vi "Do.vi"(8 "error in (no error)":errorcluster, 9 "Events":refnum<class "Events.lvclass">, 10 "Message Loop Data in":T1, 11 "IInternalRequest in":refnum<class "RegisteredHandler JSON.lvclass">) -> (0 "error out":errorcluster, 2 "Message Loop Data out":T1, 3 "IInternalRequest out":refnum<class "RegisteredHandler JSON.lvclass">)   [LabVIEW 2020, in "wamplv.lvlib" / "RegisteredHandler JSON.lvclass"]
uses:
  RegisteredHandler JSON.lvclass
  WAMP Client/Private/TypeDef/Publish Requests Map.ctl
  wamplv.lvlib
  WAMP Client/Private/TypeDef/Endpoint Data.ctl
  Call/ICallRequest/ICallRequest.lvclass
  WAMP Client/Private/TypeDef/CALL Request Map.ctl
  WAMP Client/Private/TypeDef/SUBSCRIBE Requests Map.ctl
  WAMP Client/Private/TypeDef/Subscriptions Map.ctl
  WAMP Client/Private/TypeDef/Unsubscribe Requests Map.ctl
  WAMP Client/Private/TypeDef/Unregister requests map.ctl
  WAMP Client/Private/TypeDef/Message Loop Data.ctl
  Events/EventsParent/Events.lvclass
  Subscribe/ISubscribe/ISubscribe.lvclass
  Publish/IPublish/IPublish.lvclass
  Message loop classes/Subscription details/SubscriptionDetailsParent/SubscriptionDetailsParent.lvclass
  Unsubscribe/IUnsubscribe/IUnsubscribe.lvclass
  Register/IRegister/IRegister.lvclass
  Unregister/IUnregister/IUnregister.lvclass
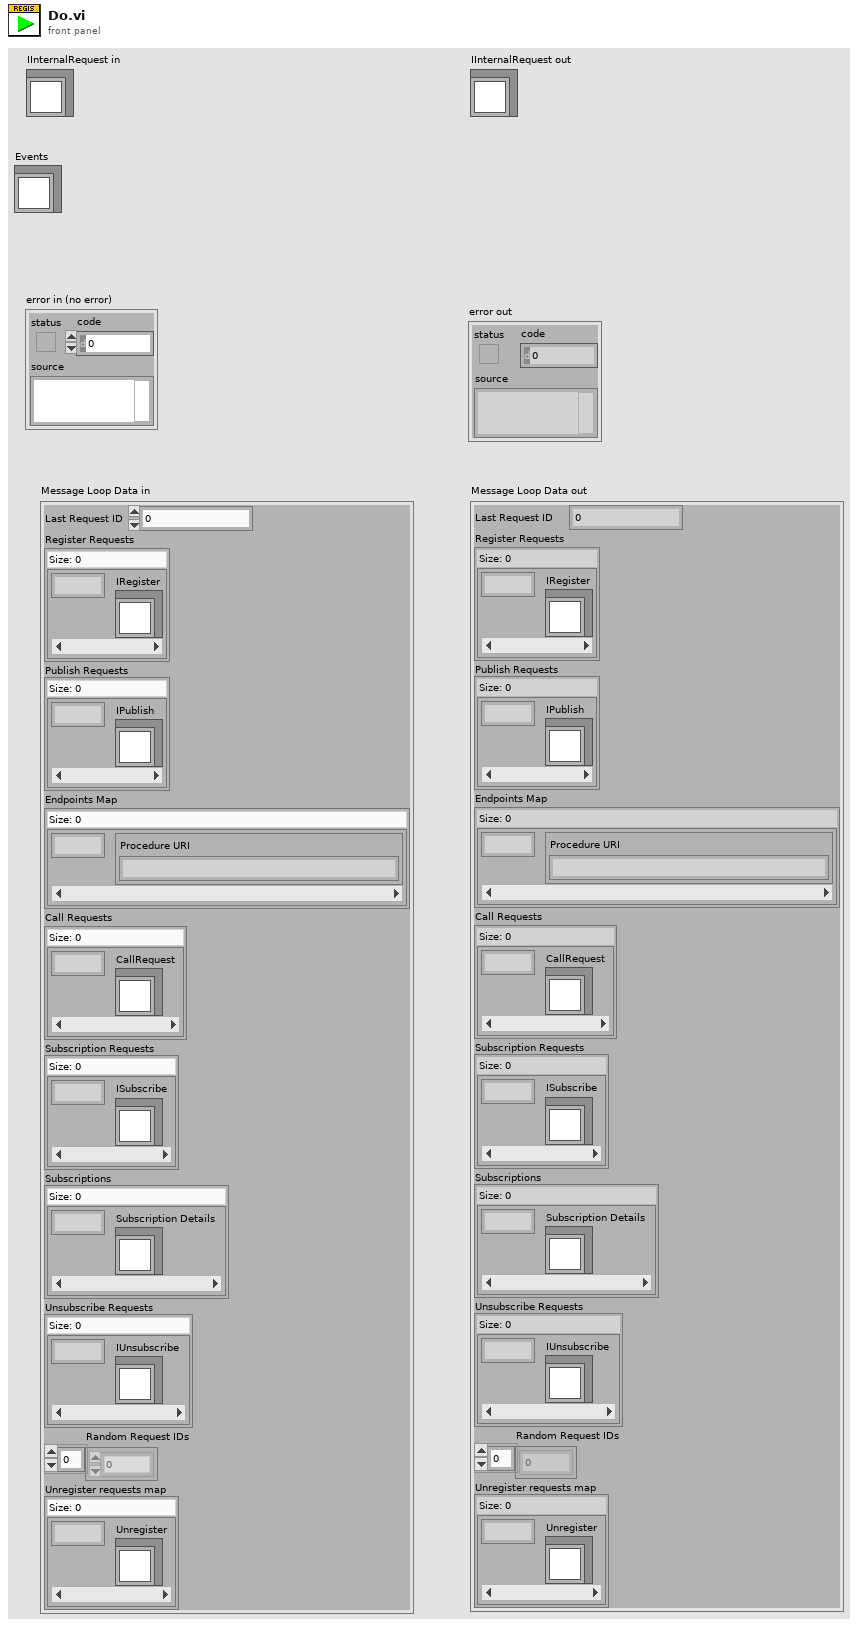
[diagram p1: front panel]
types:
  T1 = typedef "wamplv.lvlib/Message Loop Data.ctl" = cluster{"Last Request ID":u64, "Register Requests":map{u64, refnum<class "IRegister.lvclass">}, "Publish Requests":T2, "Endpoints Map":map{u64, T3}, "Call Requests":T4, "Subscription Requests":T5, "Subscriptions":T6, "Unsubscribe Requests":T7, "Random Request IDs":u64[], "Unregister requests map":T8}
  T2 = typedef "wamplv.lvlib/Publish Requests Map.ctl" = map{u64, refnum<class "IPublish.lvclass">}
  T3 = typedef "wamplv.lvlib/Endpoint Data.ctl" = cluster{"Procedure URI":string}
  T4 = typedef "wamplv.lvlib/CALL Request Map.ctl" = map{u64, refnum<class "ICallRequest.lvclass">}
  T5 = typedef "wamplv.lvlib/SUBSCRIBE Requests Map.ctl" = map{u64, refnum<class "ISubscribe.lvclass">}
  T6 = typedef "wamplv.lvlib/Subscriptions Map.ctl" = map{u64, refnum<class "SubscriptionDetailsParent.lvclass">}
  T7 = typedef "wamplv.lvlib/Unsubscribe Requests Map.ctl" = map{u64, refnum<class "IUnsubscribe.lvclass">}
  T8 = typedef "wamplv.lvlib/Unregister requests map.ctl" = map{u64, refnum<class "IUnregister.lvclass">}
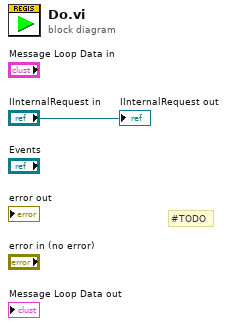
[diagram p0: block diagram]
diagram:
  # "#TODO"
  "IInternalRequest out" <- "IInternalRequest in"
